vi "CameraAndStageEnableTests.vi"() -> ()   [LabVIEW 2016]
uses:
  Motion/EnableMultiple.vi
  Motion/DisableMultiple.vi
  <vilib>/Utility/file.llb/Write Delimited Spreadsheet (DBL).vi
  <vilib>/vision/driver/NI_Vision_Acquisition_Software.lvlib
  <vilib>/vision/NI_Vision_Development_Module.lvlib
panel:
  out "STAGE IS LIVE!!":bool
  in  "file path (dialog if empty)":path
  out "current time":timestamp
  out "End time":timestamp
  in  "Measurement length [minutes]":dbl
  out "Start time":timestamp
  out "Y match pos":sgl(graph)
  out "X match pos":sgl(graph)
  in  "Pattern Match Settings":T1={"Algorithm"=2, "Number of Matches Requested"=1, "Minimum Match Score"=800.0, "SubPixel Accuracy"=TRUE, "Rotation Angle Ranges"=[{"Start"=0.0, "End"=360.0}], "Show Search Area"=FALSE, "Show Result"=TRUE} {"Rotation Angle Ranges"."End" format="%.1f"; "Rotation Angle Ranges"."Start" format="%.1f"; "Minimum Match Score" min=0 max=1000 format="%.2f"; "Number of Matches Requested" min=1; "Algorithm" items=["All", "Low Discrepancy Sampling", "Grayscale Value Pyramid", "Gradients Pyramid"]}
  in  "Template Path":path=path "C:/Users/Aerotech/Documents/BNLStaveAssembly-blueprint/image1.JPG"
  out "Y position":dbl(graph)
  out "Z position":dbl(graph)
  in  "Enable stage?":bool
  out "X position":dbl(graph)
  out "XYZ Stage Loop #":i32
  in  "Axis colour":u32(colorbox)=16711680
  out "Error report":errorcluster
  in  "stop":bool
  out "Image":T2(plugin-control) caption="Image Out"
  in  "Camera Name":refnum<k21>="cam1" caption="IMAQdx Session"
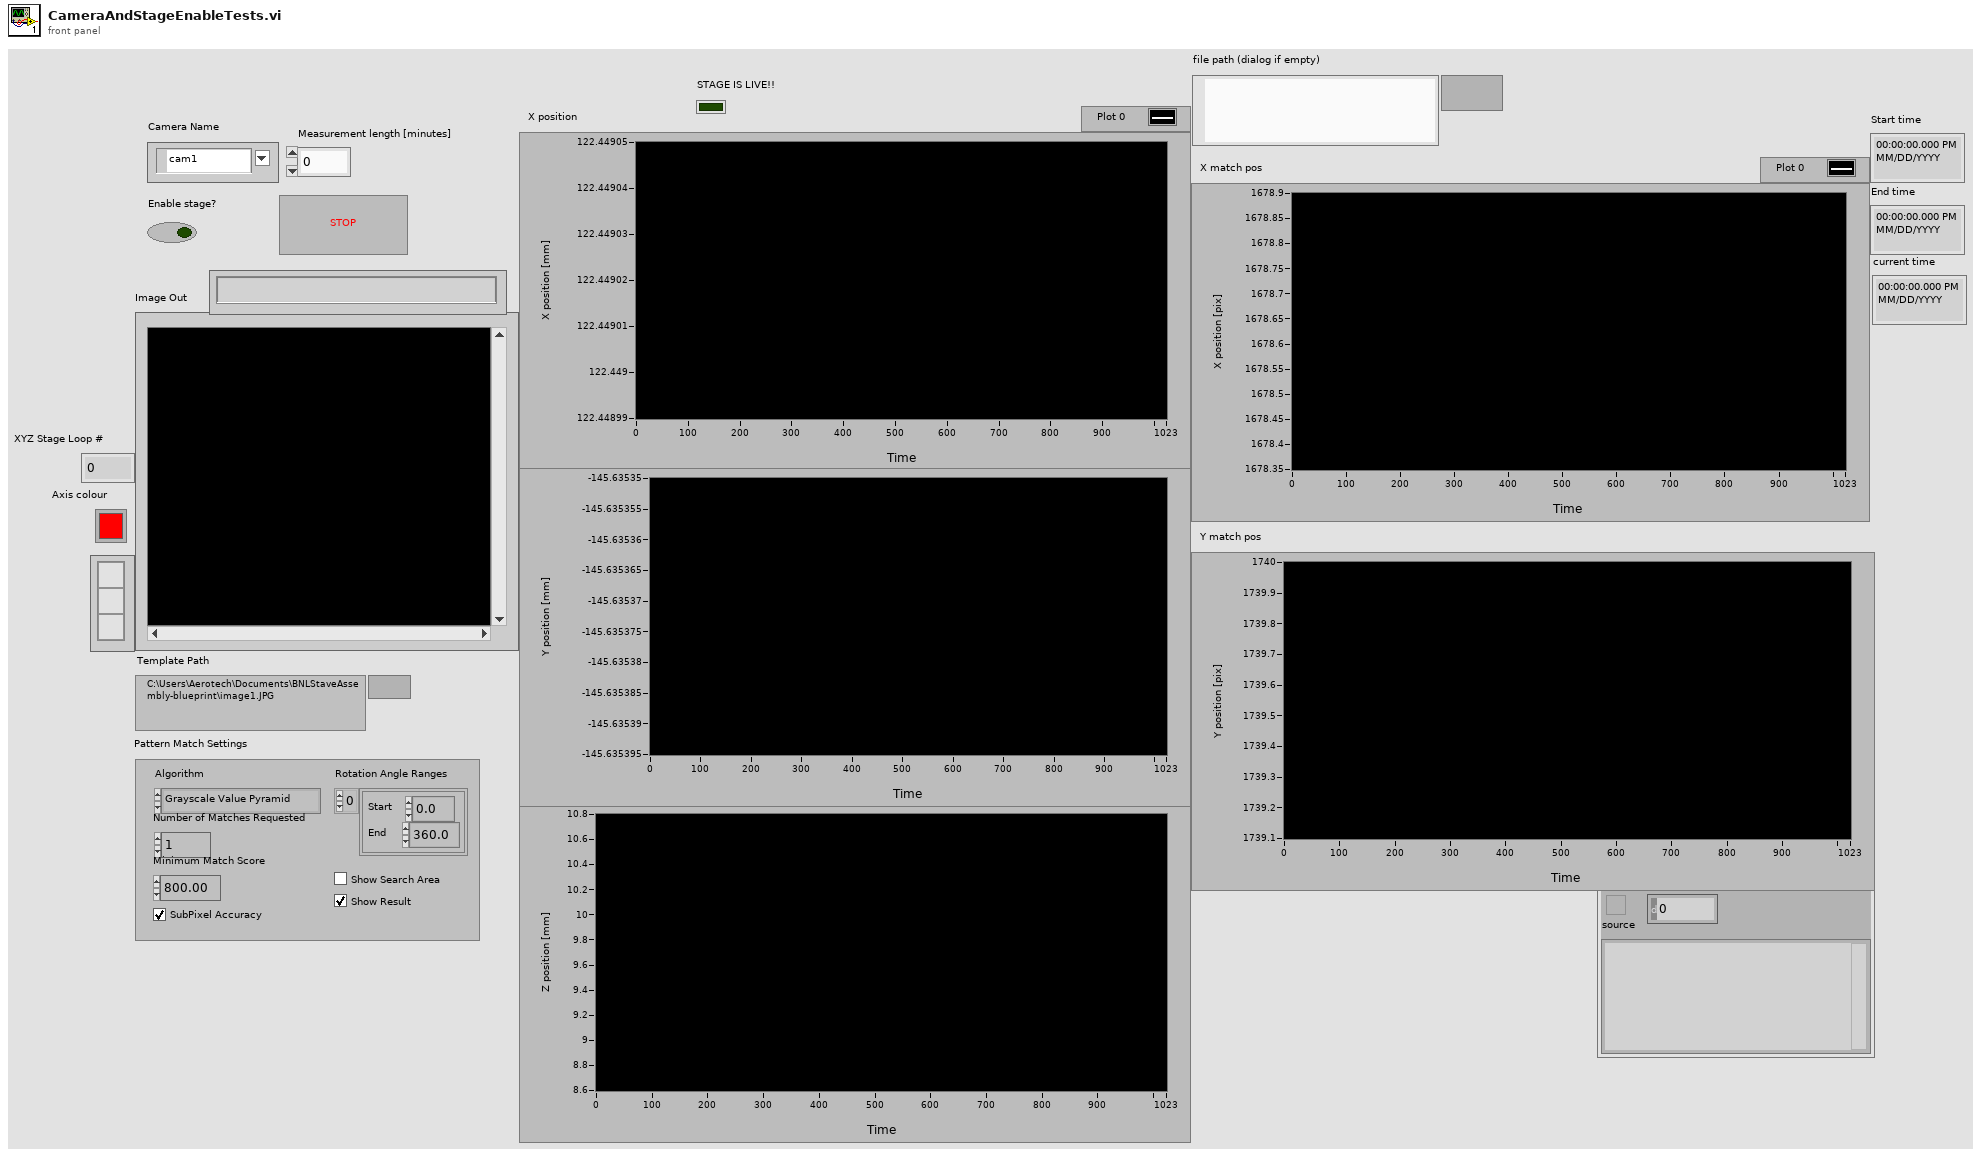
[diagram p1: front panel]
types:
  T1 = cluster{"Algorithm":i32, "Number of Matches Requested":i32, "Minimum Match Score":sgl, "SubPixel Accuracy":bool, "Rotation Angle Ranges":cluster{"Start":sgl, "End":sgl}[], "Show Search Area":bool, "Show Result":bool}
  T2 = typedef "IMAQ Image.ctl" = refnum<image>
  T3 = typedef "Image Type" = u32
  T4 = typedef "IMAQdx.ctl" = refnum<k21>
  T5 = typedef "LVDateTimeRec.ctl" = cluster{"fractional second":dbl, "second":i32, "minute":i32, "hour":i32, "day of month":i32, "month":i32, "year":i32, "day of week":i32, "day of year":i32, "DST":i32}
  T6 = cluster{"Position":cluster{"x":sgl, "y":sgl}, "Angle":sgl, "Scale":sgl, "Score":sgl, "Bounding Box":cluster{"x":sgl, "y":sgl}[]}[]
  T7 = cluster{"Position":cluster{"x":sgl, "y":sgl}, "Angle":sgl, "Scale":sgl, "Score":sgl, "Bounding Box":cluster{"x":sgl, "y":sgl}[]}
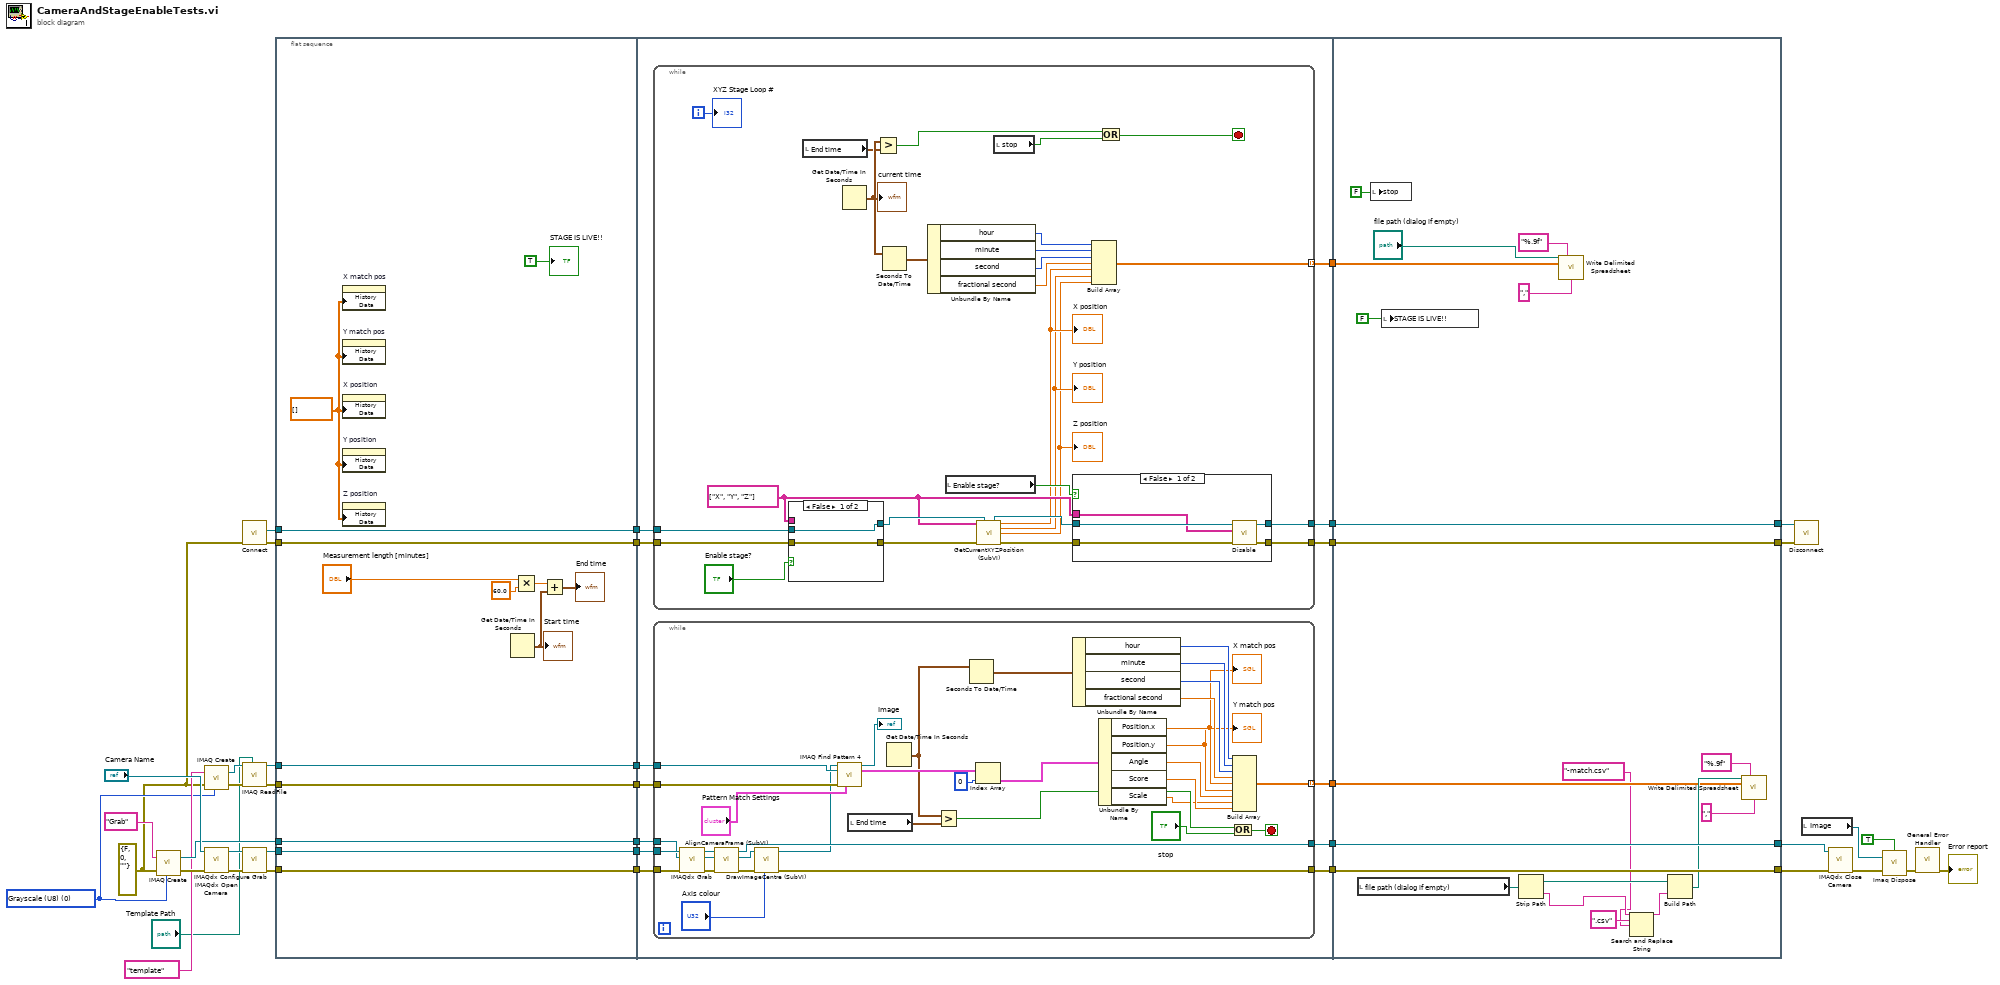
[diagram p0: block diagram]
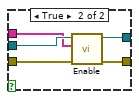
[diagram p3: hidden frame]
diagram:
  w15 = errorcluster {"status"=FALSE, "code"=0, "source"=""} ("error in (no error)")
  w16 = T3 0 items=["Grayscale (U8)", "Grayscale (I16)", "Grayscale (SGL)", "Complex (CSG)", "RGB (U32)", "HSL (U32)", "RGB (U64)", "Grayscale (U16)"] ("Image Type")
  n1 = call "IMAQ Create"("Image Name"="Grab", "Image Type"=w16, "error in (no error)"=w15) -> ("New Image"=w27:T2, "error out"=w40:errorcluster)  [unwired: 1 in, 1 out]
  n2 = call "IMAQ Create"("Image Name"="template", "Image Type"=w16, "error in (no error)"=w15) -> ("New Image"=w13:T2, "error out"=w14:errorcluster)  [unwired: 2 in]
  n3 = call <vilib>:"IMAQdx Open Camera.vi"("error in"=w40, "Session In"="Camera Name") -> ("error out"=w37:errorcluster, "Session Out"=w38:T4)  [unwired: 1 in, 7 out]
  n4 = call "Connect.vi"("error in (no error)"=w15) -> ("error out"=w24:errorcluster, "controller"=w25:refnum<k24>)  [unwired: 9 in]
  n5 = call "IMAQ ReadFile"("File Path"="Template Path", "error in (no error)"=w14, "Image"=w13) -> ("error out"=w10:errorcluster, "Image Out"=w11:T2)  [unwired: 4 in, 3 out]
  n6 = call <vilib>:"IMAQdx Configure Grab.vi"("error in"=w37, "Session In"=w38) -> ("error out"=w35:errorcluster, "Session Out"=w34:T4)  [unwired: 8 out]
  n7 = flat-sequence {
    tunnel: w10 -> [w48]
    tunnel: w11 -> [w49]
    tunnel: w24 -> [w50]
    tunnel: w25 -> [w51]
    tunnel: w27 -> [w52]
    tunnel: w34 -> [w53]
    tunnel: w35 -> [w54]
    tunnel: [w54] -> w8
    tunnel: [w53] -> w7
    tunnel: [w52] -> w6
    tunnel: [w51] -> w5
    tunnel: [w50] -> w4
    tunnel: [w49] -> w3
    tunnel: [w48] -> w2
    tunnel: [w65] -> w26
    tunnel: [w61] -> w23
    tunnel: [w60] -> w21
    tunnel: [w59] -> w19
    tunnel: [w56] -> w9
    tunnel: w8 -> [w67]
    tunnel: w7 -> [w66]
    tunnel: w6 -> [w64]
    tunnel: w5 -> [w63]
    tunnel: w4 -> [w62]
    tunnel: w3 -> [w58]
    tunnel: w2 -> [w57]
    tunnel: [w55] -> w1
    tunnel: [w162] -> w33
    tunnel: w26 -> [w162]
    tunnel: [w160] -> w22
    tunnel: w23 -> [w160]
    tunnel: w21 -> [w159]
    tunnel: [w159] -> w20
    tunnel: w19 -> [w158]
    tunnel: [w158] -> w18
    tunnel: w9 -> [w157]
    tunnel: w1 -> [w148]
    frame #0 {
      w42 = dbl[] [] ("History Data")
      n8 = property on="X match pos" class="WFChart (strict)"("History Data"=w42) -> ()  [unwired: 2 in, 2 out]
      n9 = property on="Y match pos" class="WFChart (strict)"("History Data"=w42) -> ()  [unwired: 2 in, 2 out]
      n10 = property on="X position" class="WFChart (strict)"("History Data"=w42) -> ()  [unwired: 2 in, 2 out]
      n11 = property on="Y position" class="WFChart (strict)"("History Data"=w42) -> ()  [unwired: 2 in, 2 out]
      n12 = property on="Z position" class="WFChart (strict)"("History Data"=w42) -> ()  [unwired: 2 in, 2 out]
      n13 = Get Date/Time In Seconds() -> (seconds since 1Jan1904=w46:timestamp)
      "Start time" <- w46
      n14 = Multiply(x="Measurement length [minutes]", y=60.0) -> (x*y=w45:dbl)
      n15 = Add(x=w45, y=w46) -> (x+y=→"End time":timestamp)
      "STAGE IS LIVE!!" <- TRUE ("STAGE IS LIVE!!")
    }
    frame #1 {
      n16 = while {
        tunnel: w63 -> [w92]
        tunnel: w62 -> [w91]
        tunnel: [w86] -> w61
        tunnel: [w83] -> w60
        tunnel: [w76] -> w56 mode=indexing
        i -> [w93]
        stop <- w81 stop-if-true
        w85 = string[] ["X", "Y", "Z"] ("Axes Names")
        n17 = case shown="False" "Enable stage?" {
          tunnel: w92 -> [w102 w107]
          tunnel: w85 -> [_ w106]
          tunnel: w91 -> [w101 w105]
          tunnel: [w102 w104] -> w90
          tunnel: [w101 w103] -> w89
          frame False {
          }
          frame True {
            n18 = call-poly "Enable.vi"("error in (no error)"=w105, "axis names"=w106, "controller in"=w107) -> ("error out"=w103:errorcluster, "controller out"=w104:refnum<k24>)  [unwired: 7 in]
          }
        }
        n19 = local read "End time"() -> (w68:timestamp)
        n20 = Get Date/Time In Seconds() -> (seconds since 1Jan1904=w74:timestamp)
        "current time" <- w74
        n21 = Greater?(x=w74, y=w68) -> (0:w80:bool)
        n22 = Seconds To Date/Time(time stamp (now)=w74) -> (date time rec=w73:T5)  [unwired: 1 in]
        n23 = Unbundle By Name(w73) -> ("hour"=w72:i32, "minute"=w71:i32, "second"=w70:i32, "fractional second"=w69:dbl)
        n24 = local read "Enable stage?"() -> (w88:bool)
        n25 = call "GetCurrentXYZPosition (SubVI).vi"("Axes Names"=w85, ".NET Refnum in - Device"=w90, "error in (no error)"=w89) -> (".NET Refnum out  - Device"=w87:refnum<k24>, "X Position Feedback"=w79:dbl, "Y Position Feedback"=w78:dbl, "Z Position Feedback"=w77:dbl, "error out"=w84:errorcluster)  [unwired: 7 in, 1 out]
        "X position" <- w79
        "Z position" <- w77
        "Y position" <- w78
        n26 = local read "stop"() -> (w75:bool)
        n27 = case shown="False" w88 {
          tunnel: w87 -> [w98 w99]
          tunnel: [w97 w99] -> w86
          tunnel: w85 -> [w96 _]
          tunnel: w84 -> [w95 w100]
          tunnel: [w94 w100] -> w83
          frame False {
            n28 = call-poly "Disable.vi"("error in (no error)"=w95, "axis names"=w96, "controller in"=w98) -> ("error out"=w94:errorcluster, "controller out"=w97:refnum<k24>)  [unwired: 7 in]
          }
          frame True {
          }
        }
        n29 = Build Array(w72, w71, w70, w69, w79, w78, w77) -> (w76:dbl[])
        n30 = Or(x=w80, y=w75) -> (x .or. y?=w81:bool)
        "XYZ Stage Loop #" <- w93
      }
      n31 = while {
        tunnel: w67 -> [w139]
        tunnel: w66 -> [w138]
        tunnel: [w137] -> w65
        tunnel: w64 -> [w136]
        tunnel: [w132] -> w59
        tunnel: w58 -> [w131]
        tunnel: w57 -> [w130]
        tunnel: [w109] -> w55 mode=indexing
        stop <- w123 stop-if-true
        n32 = call <vilib>:"IMAQdx Grab.vi"("error in"=w139, "Image In"=w136, "Session In"=w138) -> ("error out"=w140:errorcluster, "Image Out"=w142:T2, "Session Out"=w141:T4)  [unwired: 1 in, 5 out]
        n33 = call "AlignCameraFrame (SubVI).vi"("error in (no error)"=w140, "Image Src"=w142, "Refnum in"=w141) -> ("error out"=w133:errorcluster, "Image Dst Out"=w135:T2, "Refnum out"=w137:T4)  [unwired: 6 in]
        n34 = call "DrawImageCentre (SubVI).vi"("Axis colour"="Axis colour", "error in (no error)"=w133, "Refnum in"=w135) -> ("error out"=w132:errorcluster, "Refnum out"=w128:T2)  [unwired: 7 in]
        n35 = call "IMAQ Find Pattern 4"("Image"=w128, "Template"=w131, "error in"=w130, "Settings"="Pattern Match Settings") -> ("Image Out"=→"Image":T2, "Matches (pixel)"=w126:T6)  [unwired: 5 in, 5 out]
        n36 = local read "End time"() -> (w122:timestamp)
        n37 = Get Date/Time In Seconds() -> (seconds since 1Jan1904=w118:timestamp)
        n38 = Greater?(x=w118, y=w122) -> (0:w121:bool)
        n39 = Seconds To Date/Time(time stamp (now)=w118) -> (date time rec=w119:T5)  [unwired: 1 in]
        n40 = Index Array(array=w126, index=0) -> (element=w124:T7)
        n41 = Unbundle By Name(w119) -> ("hour"=w117:i32, "minute"=w116:i32, "second"=w115:i32, "fractional second"=w114:dbl)
        n42 = Unbundle By Name(w124) -> ("Position.x"=w113:sgl, "Position.y"=w112:sgl, "Angle"=w111:sgl, "Score"=w110:sgl, "Scale"=w108:sgl)
        "Y match pos" <- w112
        "X match pos" <- w113
        n43 = Or(x=w121, y="stop") -> (x .or. y?=w123:bool)
        n44 = Build Array(w117, w116, w115, w114, w113, w112, w111, w108, w110) -> (w109:dbl[])
      }
    }
    frame #2 {
      n45 = local read "file path (dialog if empty)"() -> (w151:path)
      n46 = local write "stop"(FALSE ("stop")) -> ()
      n47 = local write "STAGE IS LIVE!!"(FALSE ("STAGE IS LIVE!!")) -> ()
      n48 = Strip Path(path=w151) -> (stripped path=w150:path, name=w146:string)
      n49 = call-poly <vilib>:"Write Delimited Spreadsheet.vi"("file path (dialog if empty)"="file path (dialog if empty)", "format (%.3f)"="%.9f", "2D data"=w157, "delimiter (\\t)"="," ("delimiter (\\t)")) -> ()  [unwired: 10 in, 2 out]
      n50 = Search and Replace String(input string=w146, search string=".csv", replace string="-match.csv" ("string")) -> (result string=w143:string)  [unwired: 5 in, 3 out]
      n51 = Build Path(base path=w150, name or relative path=w143) -> (appended path=w149:path)
      n52 = call-poly <vilib>:"Write Delimited Spreadsheet.vi"("file path (dialog if empty)"=w149, "format (%.3f)"="%.9f", "2D data"=w148, "delimiter (\\t)"="," ("delimiter (\\t)")) -> ()  [unwired: 10 in, 2 out]
    }
  }
  n53 = call "Disconnect.vi"("error in (no error)"=w20, "controller"=w22) -> ()  [unwired: 9 in, 1 out]
  n54 = local read "Image"() -> (w32:T2)
  n55 = call <vilib>:"IMAQdx Close Camera.vi"("error in"=w18, "Session In"=w33) -> ("error out"=w30:errorcluster)  [unwired: 9 out]
  n56 = call "Imaq Dispose"("All Images? (No)"=TRUE, "Image"=w32, "error in (no error)"=w30) -> ("error out"=w29:errorcluster)  [unwired: 3 in]
  n57 = call <vilib>:"General Error Handler.vi"("error in (no error)"=w29) -> ("error out"=→"Error report":errorcluster)  [unwired: 2 in, 12 out]
